vi "CreateReferences.vi"(7 "Coorinate System?":bool, 8 "error in (no error)":errorcluster, 9 "AxisArray_FromConf":string[](array[string]), 10 "Axis Name":string="Axis 1", 11 "SoftmotionAxis in":refnum<class "SoftmotionAxis.lvclass">) -> (0 "error out":errorcluster, 3 "SoftmotionAxis out":refnum<class "SoftmotionAxis.lvclass">)   [LabVIEW 2017, in "SoftmotionAxis.lvclass"]
uses:
  SoftmotionAxis.lvclass
  <vilib>/Motion/PropertyNodes/nimc.createStraightLineMoveInstance.axis.vi
  <vilib>/Motion/PropertyNodes/nimc.createReferenceMoveInstance.axis.vi
  <vilib>/Motion/PropertyNodes/nimc.createStopMoveInstance.axis.vi
  <vilib>/Motion/PropertyNodes/nimc.destroyInterfaceInstance.vi
  <vilib>/Motion/PropertyNodes/nimc.createStraightLineMoveInstance.coordinate.vi
  <vilib>/Motion/PropertyNodes/nimc.createStopMoveInstance.coordinate.vi
  <resource>/objmgr/nimcai.rc
  <resource>/objmgr/nimotion.rc
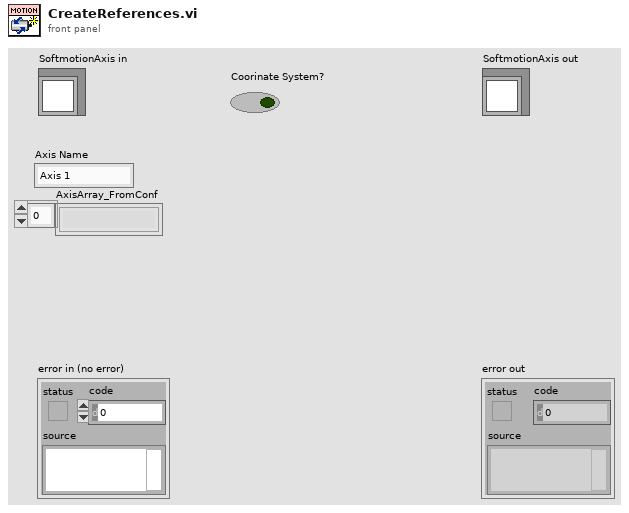
[diagram p1: front panel]
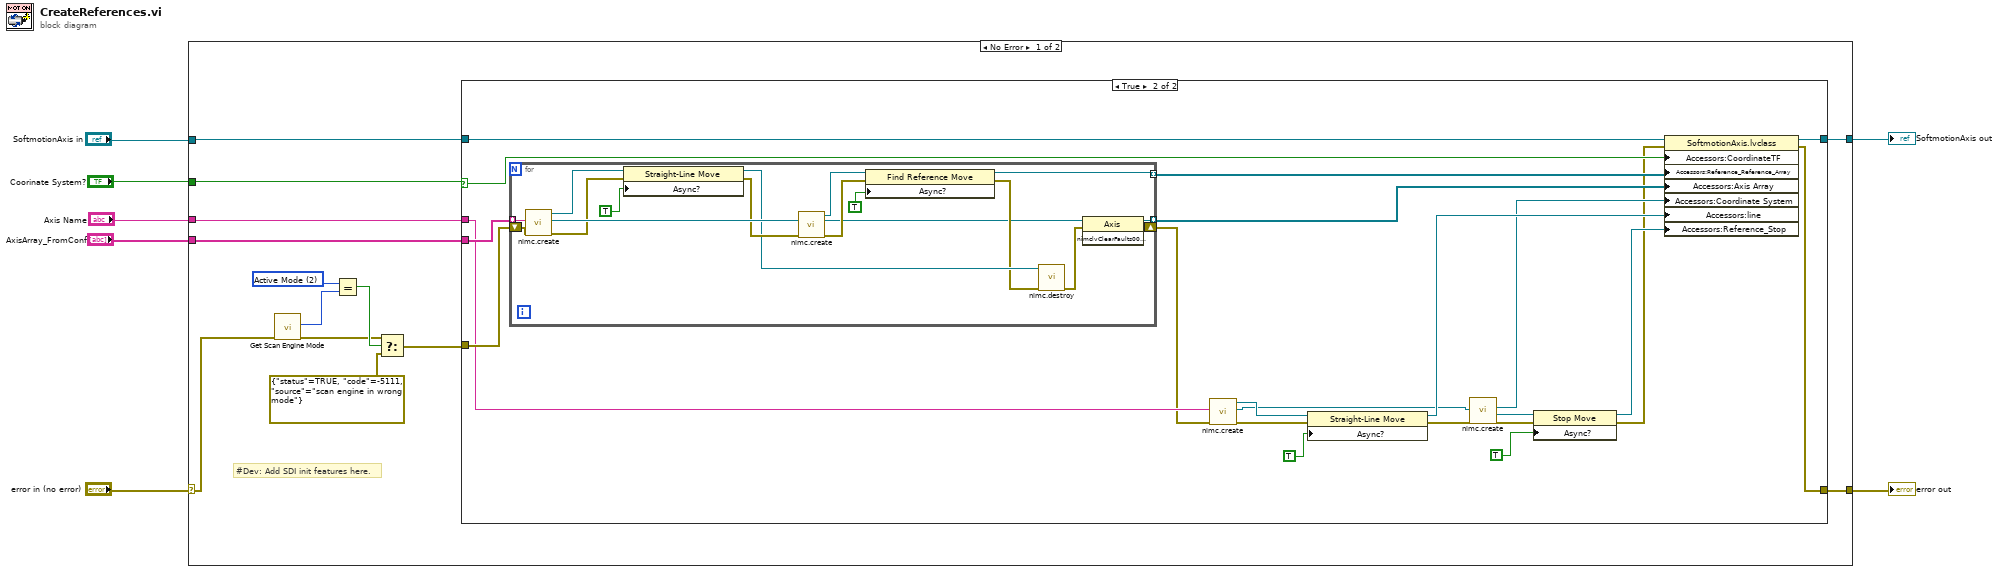
[diagram p0: block diagram]
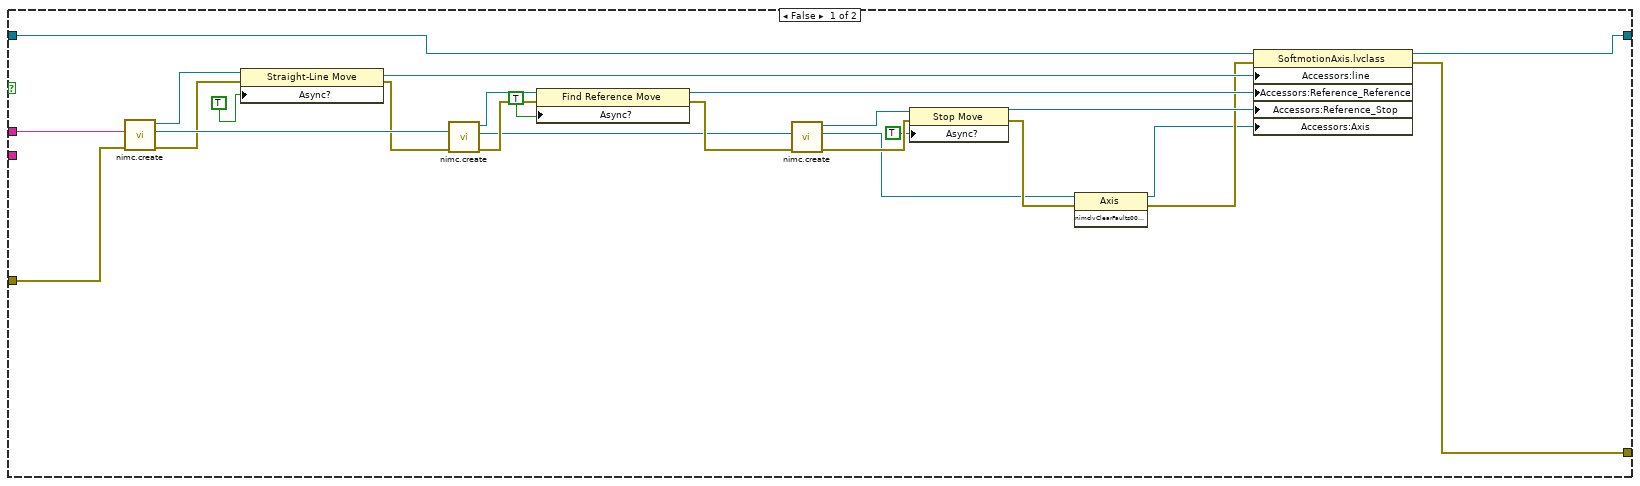
[diagram p2: hidden frame]
diagram:
  n1 = case shown="No Error" "error in (no error)" {
    selector: "error in (no error)" -> [w18 w86]
    tunnel: [w17 w86] -> w6
    tunnel: [w19 w85] -> w4
    tunnel: "SoftmotionAxis in" -> [w15 w85]
    tunnel: "Axis Name" -> [w16 _]
    tunnel: "Coorinate System?" -> [w9 _]
    tunnel: "AxisArray_FromConf" -> [w8 _]
    frame No Error {
      w13 = 2 items=["Configuration Mode"=1, "Active Mode"=2] ("mode (Active Mode)")
      # "#Dev: Add SDI init features here."
      n2 = call <vilib>:"Get Scan Engine Mode.vi"("error in (no error)"=w18) -> ("error out"=w11:errorcluster, "mode"=w14:i32)  [unwired: 9 in]
      n3 = Equal?(x=w13, y=w14) -> (x = y?=w12:bool)
      n4 = Select(t=w11, s=w12, f=errorcluster {"status"=TRUE, "code"=-5111, "source"="scan engine in wrong mode"} ("error in (no error)")) -> (s? t:f=w20:errorcluster)
      n5 = case shown="True" w9 {
        selector: w9 -> [_ w56]
        tunnel: w20 -> [w45 w67]
        tunnel: [w44 w66] -> w19
        tunnel: [w24 w51] -> w17
        tunnel: w16 -> [w42 w59]
        tunnel: w15 -> [w39 w65]
        tunnel: w8 -> [_ w64]
        frame False {
          n6 = call-poly <vilib>:"nimc.create.vi"("error in"=w45, "axis"=w42) -> ("error out"=w33:errorcluster, "axis out"=w41:refnum<k21>, "line"=w34:refnum<k20>)  [unwired: 7 in]
          n7 = property class="Straight-Line Move"(reference=w34, error in=w33, "Async?"=TRUE) -> (reference out=w43:refnum<k20>, error out=w40:errorcluster)
          n8 = call-poly <vilib>:"nimc.create.vi"("error in"=w40, "axis"=w41) -> ("error out"=w37:errorcluster, "axis out"=w30:refnum<k21>, "reference"=w38:refnum<k20>)  [unwired: 7 in]
          n9 = property class="Find Reference Move"(reference=w38, error in=w37, "Async?"=TRUE) -> (reference out=w36:refnum<k20>, error out=w31:errorcluster)
          n10 = call-poly <vilib>:"nimc.create.vi"("error in"=w31, "axis"=w30) -> ("error out"=w27:errorcluster, "axis out"=w22:refnum<k21>, "stop"=w28:refnum<k20>)  [unwired: 7 in]
          n11 = property class="Stop Move"(reference=w28, error in=w27, "Async?"=TRUE) -> (reference out=w29:refnum<k20>, error out=w23:errorcluster)
          n12 = invoke class="Axis" method="nimclvClearFaults00A10001"(reference=w22, error in=w23) -> (reference out=w21:refnum<k21>, error out=w25:errorcluster)  [unwired: 1 in, 1 out]
          n13 = property class="SoftmotionAxis.lvclass"(reference=w39, error in=w25, "Accessors:line"=w43, "Accessors:Reference_Reference"=w36, "Accessors:Reference_Stop"=w29, "Accessors:Axis"=w21) -> (reference out=w44:refnum<class "SoftmotionAxis.lvclass">, error out=w24:errorcluster)
        }
        frame True {
          n14 = for {
            shift-right: [w83] -> w58
            shift-left: w67 -> [w84]
            tunnel: w64 -> [w74] mode=indexing
            tunnel: [w73] -> w63 mode=indexing
            tunnel: [w72] -> w55 mode=indexing
            n15 = call-poly <vilib>:"nimc.create.vi"("error in"=w84, "axis"=w74) -> ("error out"=w76:errorcluster, "axis out"=w82:refnum<k21>, "line"=w77:refnum<k20>)  [unwired: 7 in]
            n16 = property class="Straight-Line Move"(reference=w77, error in=w76, "Async?"=TRUE) -> (reference out=w71:refnum<k20>, error out=w81:errorcluster)
            n17 = call-poly <vilib>:"nimc.create.vi"("error in"=w81, "axis"=w82) -> ("error out"=w79:errorcluster, "axis out"=w68:refnum<k21>, "reference"=w80:refnum<k20>)  [unwired: 7 in]
            n18 = property class="Find Reference Move"(reference=w80, error in=w79, "Async?"=TRUE) -> (reference out=w73:refnum<k20>, error out=w70:errorcluster)
            n19 = call-poly <vilib>:"nimc.destroy.vi"("error in"=w70, "motion handle"=w71) -> ("error out"=w69:errorcluster)  [unwired: 9 in]
            n20 = invoke class="Axis" method="nimclvClearFaults00A10001"(reference=w68, error in=w69) -> (reference out=w72:refnum<k21>, error out=w83:errorcluster)  [unwired: 1 in, 1 out]
          }
          n21 = call-poly <vilib>:"nimc.create.vi"("error in"=w58, "coordinate"=w59) -> ("error out"=w61:errorcluster, "coordinate out"=w54:refnum<k21>, "line"=w60:refnum<k20>)  [unwired: 7 in]
          n22 = property class="Straight-Line Move"(reference=w60, error in=w61, "Async?"=TRUE) -> (reference out=w57:refnum<k20>, error out=w52:errorcluster)
          n23 = call-poly <vilib>:"nimc.create.vi"("error in"=w52, "coordinate"=w54) -> ("error out"=w47:errorcluster, "coordinate out"=w53:refnum<k21>, "stop"=w49:refnum<k20>)  [unwired: 7 in]
          n24 = property class="Stop Move"(reference=w49, error in=w47, "Async?"=TRUE) -> (reference out=w48:refnum<k20>, error out=w46:errorcluster)
          n25 = property class="SoftmotionAxis.lvclass"(reference=w65, error in=w46, "Accessors:CoordinateTF"=w56, "Accessors:Reference_Reference_Array"=w63, "Accessors:Axis Array"=w55, "Accessors:Coordinate System"=w53, "Accessors:line"=w57, "Accessors:Reference_Stop"=w48) -> (reference out=w66:refnum<class "SoftmotionAxis.lvclass">, error out=w51:errorcluster)
        }
      }
    }
    frame Error {
    }
  }
  "error out" <- w6
  "SoftmotionAxis out" <- w4
